vi "Send Mail.vi"(1 "Recipient's Email Address":string, 2 "Message":string) -> ()   [LabVIEW 2016]
panel:
  in  "Enable SSL":bool
  in  "Password":string="jMli5nE!"
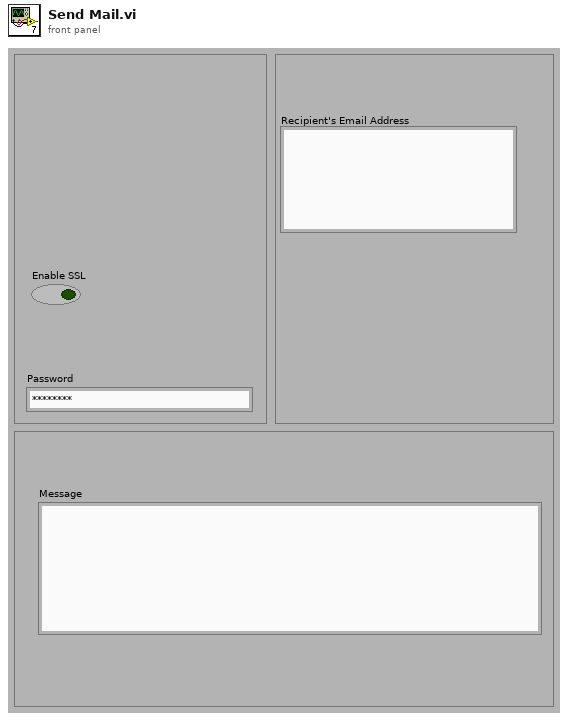
[diagram p1: front panel]
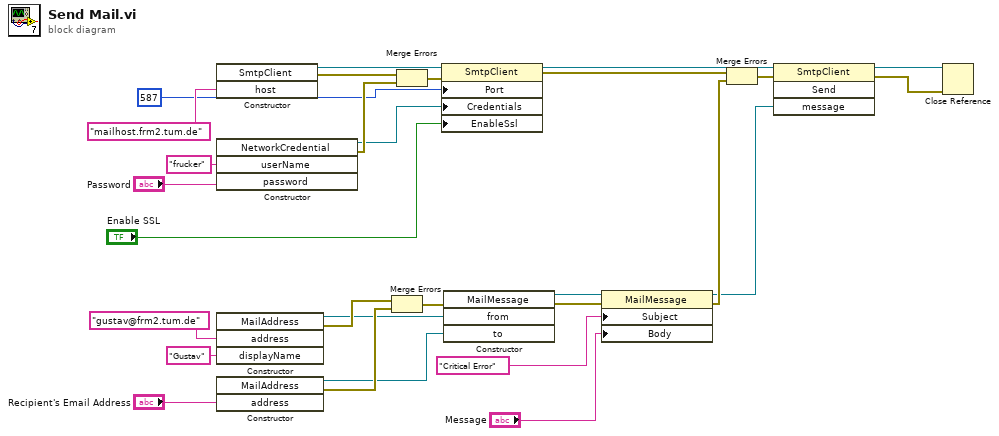
[diagram p0: block diagram]
diagram:
  n1 = constructor class="SmtpClient"("host"="mailhost.frm2.tum.de" ("SMTP Server")) -> (reference out=w11:refnum<k24>, error out=w21:errorcluster)  [unwired: 3 in, 2 out]
  n2 = constructor class="NetworkCredential"("userName"="frucker" ("Username"), "password"="Password") -> (reference out=w16:refnum<k24>, error out=w22:errorcluster)  [unwired: 3 in, 3 out]
  n3 = constructor class="MailAddress"("address"="gustav@frm2.tum.de" ("Sender's Email Address"), "displayName"="Gustav" ("Sender's Name")) -> (reference out=w2:refnum<k24>, error out=w28:errorcluster)  [unwired: 3 in, 3 out]
  n4 = constructor class="MailAddress"("address"="Recipient's Email Address") -> (reference out=w1:refnum<k24>, error out=w29:errorcluster)  [unwired: 3 in, 2 out]
  n5 = Merge Errors(w28, w29) -> (w27:errorcluster)
  n6 = Merge Errors(w21, w22) -> (w20:errorcluster)
  n7 = property class="SmtpClient"(reference=w11, error in=w20, "Port"=587, "Credentials"=w16, "EnableSsl"="Enable SSL") -> (reference out=w18:refnum<k24>, error out=w24:errorcluster)
  n8 = constructor class="MailMessage"(error in=w27, "from"=w2, "to"=w1) -> (reference out=w7:refnum<k24>, error out=w26:errorcluster)  [unwired: 2 in, 3 out]
  n9 = property class="MailMessage"(reference=w7, error in=w26, "Subject"="Critical Error", "Body"="Message") -> (reference out=w19:refnum<k24>, error out=w25:errorcluster)
  n10 = Merge Errors(w24, w25) -> (w23:errorcluster)
  n11 = invoke class="SmtpClient" method="Send"(reference=w18, error in=w23, "message"=w19) -> (reference out=w10:refnum<k24>, error out=w9:errorcluster)  [unwired: 1 in, 2 out]
  n12 = Close Reference(reference=w10, error in (no error)=w9) -> ()  [unwired: 1 out]
